vi "CreateSelfReference.vi"(8 "error in (no error)":errorcluster, 11 "SMO":refnum<class "SMO.lvclass">) -> (0 "error out":errorcluster, 3 "SMO out":refnum<class "SMO.lvclass">)   [LabVIEW 2021, in "smo.lvlib" / "SMO.lvclass"]
uses:
  SMO.lvclass
  SMO.lvclass/SMO.ctl
  Typedefs/Process Error Notification--Cluster.ctl
  Typedefs/SMOState --Enum.ctl
panel:
  # "For instructions on how to use the JKI State Machine Objects, examples and video tutorials, visit:\nhttp://jki.net/state-machine-objects/\n\nJKI State Machine Objects™\nhttp://jki.net/state-machine-objects/\nCopyright (C) 2005-2015, JKI <info@jki.net>\nALL RIGHTS RESERVED"
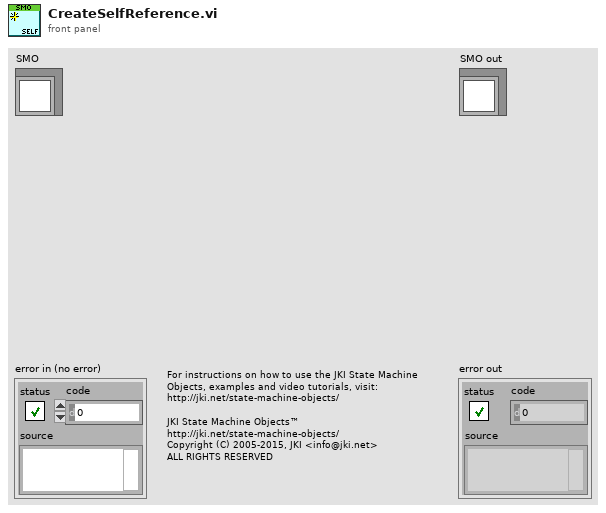
[diagram p1: front panel]
types:
  T1 = typedef "smo.lvlib/SMO.lvclass/PrivateData--Ref.ctl" = refnum<data-value>
  T2 = typedef "smo.lvlib/SMO.lvclass/PrivateData--Cluster.ctl" = cluster{"Parent Call":T3, "Registered Processes":T4[], "Sync Notifier":refnum<notifier>, "Process Error Notifier":refnum<notifier>, "Protected Events":T5, "Public Events":T6, "SMO State":T7, "[Attributes]":variant, "Launcher Close":refnum<notifier>, "Caller Watchdog":refnum<queue>, "Accessibility":T8, "NbStaticDependencies":u32}
  T3 = typedef "smo.lvlib/SMO.lvclass/Parent Call--Enum.ctl" = enum16{"Allows parent to run", "Does not request parent to run"}
  T4 = typedef "smo.lvlib/SMO.lvclass/RegisteredProcessData--Cluster.ctl" = cluster{"Name":string, "Static VI Ref":refnum<vi>, "Running":bool, "NotifierRef":u32}
  T5 = typedef "smo.lvlib/SMO.lvclass/Protected Events.ctl" = cluster{"StopProcesses":refnum<user-event>, "AbortProcesses":refnum<user-event>, "Config Changed":refnum<user-event>, "Dependency":refnum<user-event>}
  T6 = typedef "smo.lvlib/SMO.lvclass/Public Events.ctl" = cluster{"Error":refnum<user-event>, "State":refnum<user-event>, "Reserve State":refnum<user-event>}
  T7 = typedef "smo.lvlib/SMO.lvclass/SMOState --Enum.ctl" = enum16{"unknown", "Created", "Started", "Stopped"}
  T8 = typedef "smo.lvlib/SMO.lvclass/Accessibility--Cluster.ctl" = cluster{"Lock Key":string, "Reserve State":T9}
  T9 = typedef "smo.lvlib/SMO.lvclass/Reserve State--Enum.ctl" = enum16{"Unreserved", "Reserved", "Self-locked"}
  T10 = typedef "smo.lvlib/SMO.lvclass/Process Error Notification--Cluster.ctl" = cluster{"error":errorcluster}
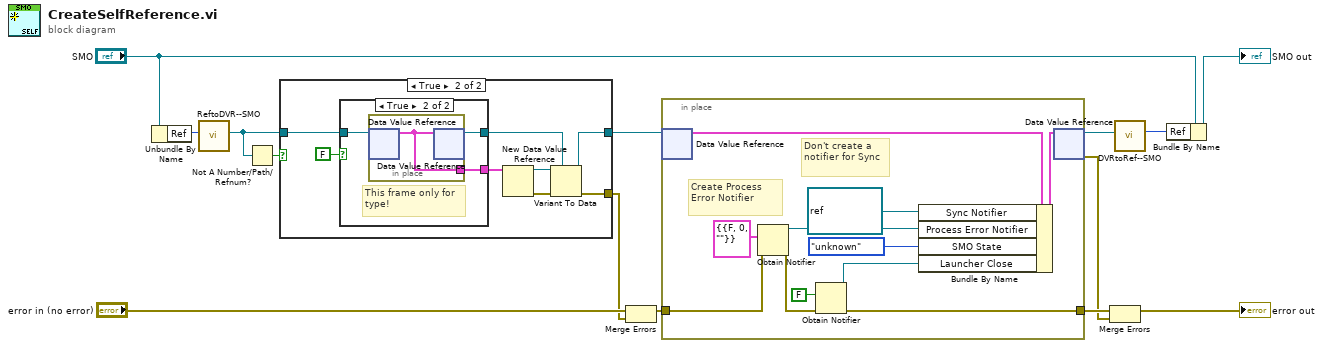
[diagram p0: block diagram]
diagram:
  n1 = Unbundle By Name("SMO") -> ("Ref"=w12:u32)
  n2 = call "ReftoDVR--SMO.vi"("Ref"=w12) -> ("Ref"=w8:T1)  [unwired: 10 in]
  n3 = Not A Number/Path/Refnum?(number/path/refnum=w8) -> (NaN/Path/Refnum?=w7:bool)
  n4 = case shown="True" w7 {
    tunnel: [w15 w17] -> w9
    tunnel: w8 -> [w15 w21]
    tunnel: [_ w16] -> w6
    frame False {
    }
    frame True {
      n5 = case shown="True" FALSE {
        tunnel: [_ w27] -> w23
        tunnel: w21 -> [w24 w26]
        tunnel: [w24 w25] -> w20
        frame False {
        }
        frame True {
          # "This frame only for\ntype!"
          n6 = in-place {
            in-place-border: [w28] -> w27
            n7 = in-place-dvr #1(w26) -> (w28:T2)  [unwired: 1 out]
            n8 = in-place-dvr #1(w28) -> (w25:T1)  [unwired: 1 out]
          }
        }
      }
      n9 = New Data Value Reference(data value=w23) -> (data value reference=w18:refnum<data-value>, error out=w19:errorcluster)  [unwired: 1 in]
      n10 = Variant To Data(error in=w19, type=w20, Variant=w18) -> (data=w17:T1, error out=w16:errorcluster)
    }
  }
  n11 = Merge Errors("error in (no error)", w6) -> (w5:errorcluster)
  n12 = in-place {
    in-place-border: [w30] -> w11
    in-place-border: w5 -> [w35]
    # "Don't create a notifier for Sync"
    # "Create Process Error Notifier"
    n13 = in-place-dvr #2(w9) -> (w39:T2)  [unwired: 1 out]
    n14 = Obtain Notifier(notification data type=T10 {"error"={"status"=FALSE, "code"=0, "source"=""}} ("Process Notification"), error in (no error)=w35) -> (notifier out=w37:refnum<notifier>, error out=w31:errorcluster)  [unwired: 2 in, 1 out]
    n15 = Obtain Notifier(notification data type=FALSE ("Launcher Close"), error in (no error)=w31) -> (notifier out=w29:refnum<notifier>, error out=w30:errorcluster)  [unwired: 2 in, 1 out]
    n16 = Bundle By Name(cluster=w39, "Sync Notifier"=refnum<notifier> refnum, "Process Error Notifier"=w37, "SMO State"=SMOState_--Enum."unknown", "Launcher Close"=w29) -> (w38:T2)
    n17 = in-place-dvr #2(w38) -> (w4:T1, w10:errorcluster)
  }
  n18 = Merge Errors(w11, w10) -> (→"error out":errorcluster)
  n19 = call "DVRtoRef--SMO.vi"("Ref"=w4) -> ("Ref"=w3:u32)  [unwired: 10 in]
  n20 = Bundle By Name(cluster="SMO", "Ref"=w3) -> (→"SMO out":refnum<class "SMO.lvclass">)
